vi "生成-剂量率报警记录数据文件-网络版.vi"(9 "缓存绘图数据":T1, 11 "探测器信息":T2) -> ()   [LabVIEW 2017]
uses:
  <vilib>/gmath/NI_Gmath.lvlib
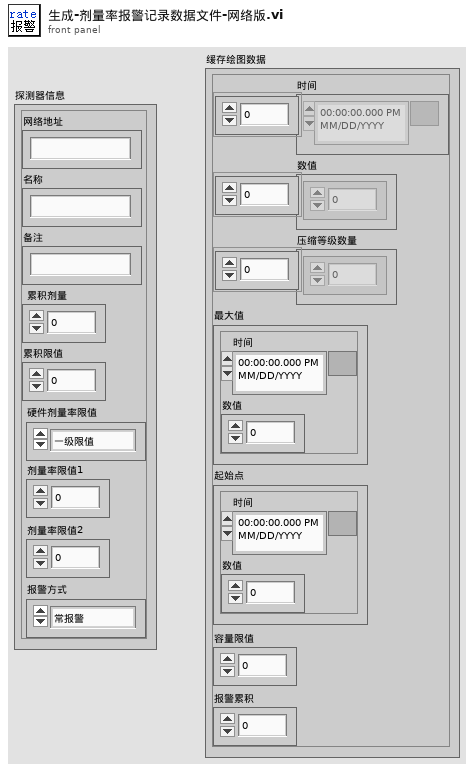
[diagram p1: front panel]
types:
  T1 = typedef "时值缓存压缩模块.lvlib/缓存数据.ctl" = cluster{"时间":timestamp[], "数值":dbl[], "压缩等级数量":i32[], "最大值":cluster{"时间":timestamp, "数值":dbl}, "起始点":cluster{"时间":timestamp, "数值":dbl}, "容量限值":i32, "报警累积":dbl}
  T2 = typedef "探测器信息.ctl" = cluster{"网络地址":string, "名称":string, "备注":string, "累积剂量":dbl, "累积限值":dbl, "硬件剂量率限值":T3, "剂量率限值1":dbl, "剂量率限值2":dbl, "报警方式":T4}
  T3 = typedef "探头剂量率限值选择.ctl" = enum16{"一级限值", "二级限值"}
  T4 = typedef "报警方式选择.ctl" = enum16{"常报警", "自动静音", "手动静音"}
  T5 = cluster{"起始时间":timestamp, "数值(rate/dose)":dbl, "报警累积":dbl}
  T6 = typedef "探头状态.ctl" = enum16{"正常", "离线", "禁用", "一级报警", "二级报警", "累积报警"}
  T7 = typedef "通用报警记录.ctl" = cluster{"探头状态":T6, "探头地址与信息":T2, "缓存绘图数据":T1, "平均值":dbl, "报警时长":cluster{"分":u16, "秒":u16}, "结论":string}
  T8 = enum16{"arithmetic", "geometric", "harmonic", "trimmed", "median"}
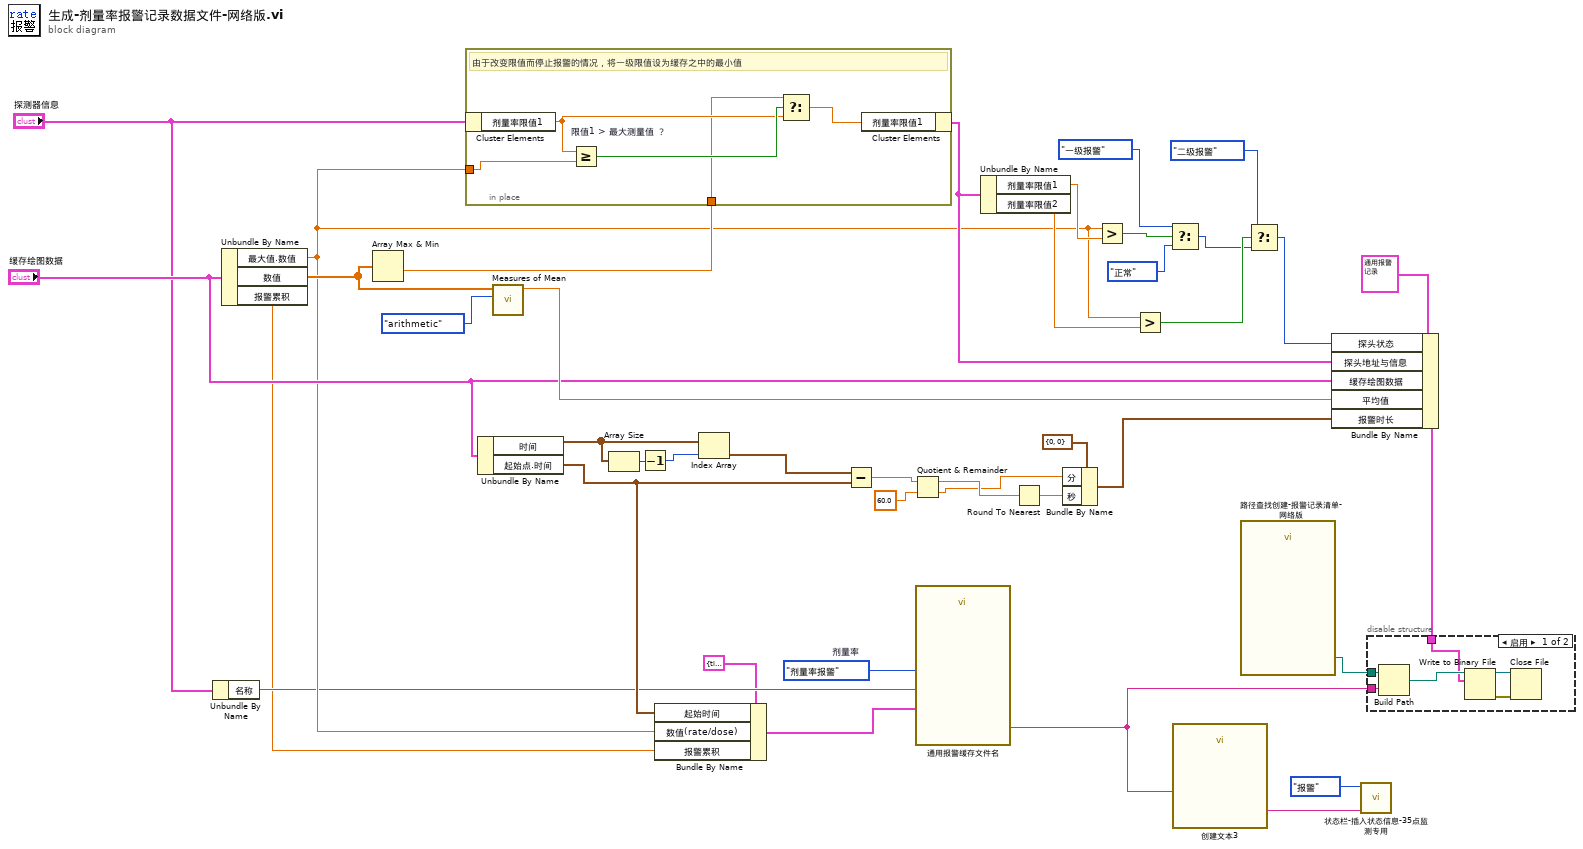
[diagram p0: block diagram]
diagram:
  w8 = enum16{"剂量率报警", "累积剂量报警"}."剂量率报警"  # 剂量率
  n1 = Unbundle By Name("探测器信息") -> ("名称"=w4:string)
  n2 = Unbundle By Name("缓存绘图数据") -> ("最大值.数值"=w6:dbl, "数值"=w37:dbl[], "报警累积"=w2:dbl)
  n3 = Array Max & Min(array=w37) -> (min value=w35:dbl)  [unwired: 3 out]
  n4 = in-place {
    in-place-border: w6 -> [w44]
    in-place-border: w35 -> [w41]
    # "由于改变限值而停止报警的情况，将一级限值设为缓存之中的最小值"
    n5 = in-place-cluster #1("探测器信息") -> ("剂量率限值1"=w43:dbl)
    n6 = Greater Or Equal? "限值1 > 最大测量值 ？"(x=w43, y=w44) -> (x >= y?=w45:bool)
    n7 = Select(t=w41, s=w45, f=w43) -> (s? t:f=w42:dbl)
    n8 = in-place-cluster #1("剂量率限值1"=w42) -> (w25:T2)
  }
  n9 = Unbundle By Name("缓存绘图数据") -> ("时间"=w22:timestamp[], "起始点.时间"=w7:timestamp)
  n10 = call <vilib>:"Measures of Mean.vi"("type"=T8."arithmetic", "x array"=w37) -> ("mean value"=w24:dbl)  [unwired: 8 in, 1 out]
  n11 = Array Size(array=w22) -> (size(s)=w21:i32)
  n12 = Decrement(x=w21) -> (x-1=w20:i32)
  n13 = Bundle By Name(cluster=T5 {"起始时间"=timestamp(0 s since 1904-01-01), "数值(rate/dose)"=0.0, "报警累积"=0.0} ("时值"), "起始时间"=w7, "数值(rate/dose)"=w6, "报警累积"=w2) -> (w5:T5)
  n14 = Index Array(array=w22, index=w20) -> (element=w19:timestamp)
  n15 = Subtract(x=w19, y=w7) -> (x-y=w18:dbl)
  n16 = Quotient & Remainder(x=w18, y=60.0) -> (x-y*floor(x/y)=w14:dbl, floor(x/y)=w13:dbl)
  n17 = call "通用报警缓存文件名.vi"("报警类型"=w8, "时值"=w5, "名称"=w4) -> ("文件名"=w3:string)  [unwired: 8 in]
  n18 = Unbundle By Name(w25) -> ("剂量率限值1"=w34:dbl, "剂量率限值2"=w30:dbl)
  n19 = Round To Nearest(number=w14) -> (nearest integer value=w12:dbl)
  n20 = Bundle By Name(cluster=cluster{"分":u16, "秒":u16} {"分"=0, "秒"=0} ("报警时长"), "分"=w13, "秒"=w12) -> (w15:cluster{"分":u16, "秒":u16})
  n21 = Greater?(x=w6, y=w34) -> (0:w33:bool)
  n22 = Greater?(x=w6, y=w30) -> (0:w29:bool)
  n23 = Select(t=探头状态."一级报警" ("探头状态"), s=w33, f=探头状态."正常" ("探头状态")) -> (s? t:f=w28:T6)
  n24 = call "创建文本3"("文件名"=w3) -> ("Result"=w40:string)  [unwired: 13 in, 1 out]
  n25 = call "路径查找创建-报警记录清单-网络版.vi"() -> ("缓存数据文件夹"=w11:path)  [unwired: 2 in, 13 out]
  n26 = Select(t=探头状态."二级报警" ("探头状态"), s=w29, f=w28) -> (s? t:f=w26:T6)
  n27 = Bundle By Name(cluster=T7 {"探头状态"=enum."正常", "探头地址与信息"={"网络地址"="", "名称"="", "备注"="", "累积剂量"=0.0, "累积限值"=0.0, "硬件剂量率限值"=enum."一级限值", "剂量率限值1"=0.0, "剂量率限值2"=0.0, "报警方式"=enum."常报警"}, "缓存绘图数据"={"时间"=[], "数值"=[], "压缩等级数量"=[], "最大值"={"时间"=timestamp(0 s since 1904-01-01), "数值"=0.0}, "起始点"={"时间"=timestamp(0 s since 1904-01-01), "数值"=0.0}, "容量限值"=0, "报警累积"=0.0}, "平均值"=0.0, "报警时长"={"分"=0, "秒"=0}, "结论"=""} ("报警记录"), "探头状态"=w26, "探头地址与信息"=w25, "缓存绘图数据"="缓存绘图数据", "平均值"=w24, "报警时长"=w15) -> (w9:T7)
  n28 = call "状态栏-插入状态信息-35点监测专用.vi"("消息内容"=w40, "状态类型"=enum16{"全部", "报警", "通信", "设置"}."报警") -> ()  [unwired: 10 in]
  n29 = disable-structure shown="启用" {
    disable-tunnel: w11 -> [w49 _]
    disable-tunnel: w3 -> [w48 _]
    disable-tunnel: w9 -> [w46 _]
    frame Enabled {
      n30 = Build Path(base path=w49, name or relative path=w48) -> (appended path=w47:path)
      n31 = Write to Binary File(file (use dialog)=w47, data=w46) -> (refnum out=w50:refnum<file>, error out=w51:errorcluster)  [unwired: 4 in, 1 out]
      n32 = Close File(refnum=w50, error in=w51) -> ()  [unwired: 2 out]
    }
    frame Disabled {
    }
  }
